vi "A_Op Amp Limits.vi"(10 "Lead Lag":dbl) -> (0 "Controller Output":dbl, 2 "Write DAQmx":dbl)   [LabVIEW 2011]
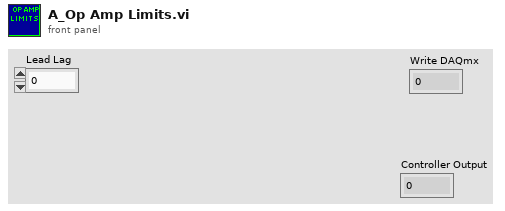
[diagram p1: front panel]
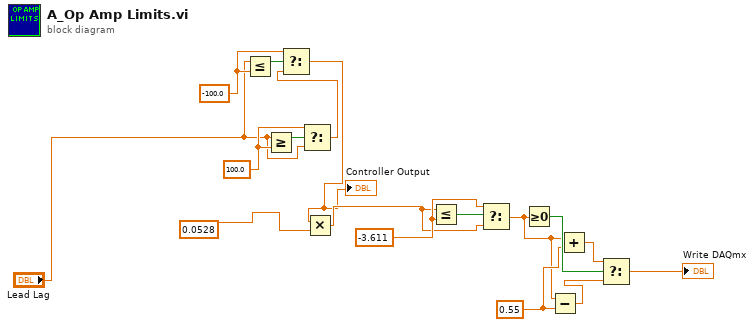
[diagram p0: block diagram]
diagram:
  w5 = -100.0 ("y")
  w10 = -3.611 ("y")
  w12 = 100.0 ("y")
  w14 = 0.55 ("y")
  n1 = Less Or Equal?(x="Lead Lag", y=w5) -> (x <= y?=w6:bool)
  n2 = Greater Or Equal?(x="Lead Lag", y=w12) -> (x >= y?=w13:bool)
  n3 = Select(t=w12, s=w13, f="Lead Lag") -> (s? t:f=w4:dbl)
  n4 = Select(t=w5, s=w6, f=w4) -> (s? t:f=w3:dbl)
  "Controller Output" <- w3
  n5 = Multiply(x=w3, y=0.0528) -> (x*y=w9:dbl)
  n6 = Less Or Equal?(x=w9, y=w10) -> (x <= y?=w11:bool)
  n7 = Select(t=w10, s=w11, f=w9) -> (s? t:f=w8:dbl)
  n8 = Greater Or Equal To 0?(x=w8) -> (x >= 0?=w17:bool)
  n9 = Subtract(x=w8, y=w14) -> (x-y=w16:dbl)
  n10 = Add(x=w8, y=w14) -> (x+y=w15:dbl)
  n11 = Select(t=w15, s=w17, f=w16) -> (s? t:f=→"Write DAQmx":dbl)
